vi "Refnums.vi"() -> ()   [LabVIEW 2015]
panel:
  in  "Bottom Limit":string="DIO1"
  in  "Top Limit":string="DIO0"
  in  "Arm":string="PWM9"
  in  "DriveL":string="DriveL"
  in  "Indexer":string="PWM8"
  in  "ShooterWheel2":string="PWM7"
  in  "ShooterWheel1":string="PWM6"
  in  "Gunner":string="Gunner"
  in  "DriveR":string="DriveR"
  in  "Left1":string="PWM3"
  in  "Left2":string="PWM4"
  in  "Left3":string="PWM5"
  in  "Right3":string="PWM2"
  in  "Right1":string="PWM0"
  in  "Right2":string="PWM1"
  # "PWM"
  # "Joystick"
  # "Drive"
  # "DIO"
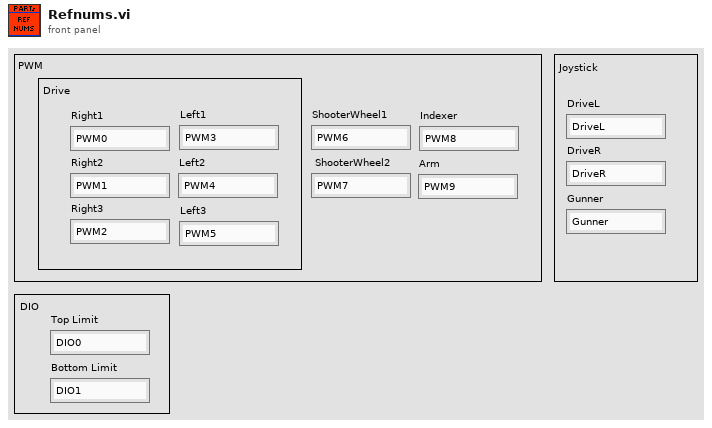
[diagram p1: front panel]
diagram:
